vi "创建数据表.vi"(8 "error in (no error)":errorcluster) -> (0 "error out":errorcluster)   [LabVIEW 2016, in "数据查询.lvlib"]
uses:
  <vilib>/addons/database/Auxilliary.llb/DB Tools Column Info.ctl
  <vilib>/addons/database/Auxilliary.llb/DB Tools DataTypes.ctl
  <vilib>/addons/database/Connection.llb/DB Tools Open Connec (String).vi
  <userlib>/_LVST/sqlite_api/Core/Tables/SQLite_Drop Table.vi
  <userlib>/_LVST/sqlite_api/Core/Tables/SQLite_Create Table.vi
  <vilib>/addons/database/NI_Database_API.lvlib
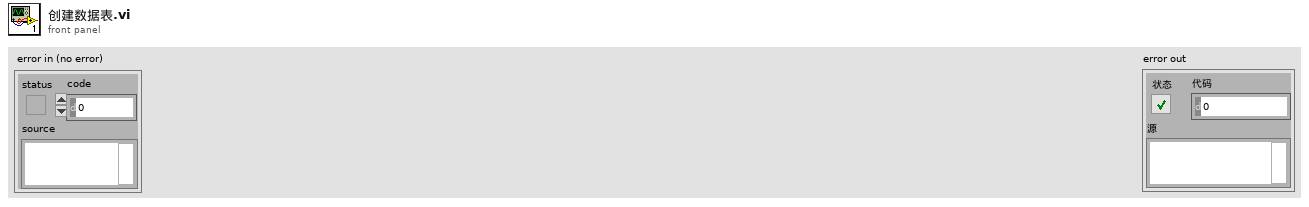
[diagram p1: front panel]
types:
  T1 = typedef "数据库类型.ctl" = enum16{"Access", "SQLite"}
  T2 = typedef "NI_Database_API.lvlib/DB Tools Column Info.ctl" = cluster{"column name":string, "data type":T3, "size":i32, "allow null?":bool}
  T3 = typedef "NI_Database_API.lvlib/DB Tools DataTypes.ctl" = enum16{"String", "Long (I32)", "Single (SGL)", "Double (DBL)", "Date/Time", "Binary"}
  T4 = typedef "NI_Database_API.lvlib/Conn ObjectReference.ctl" = refnum<k1>
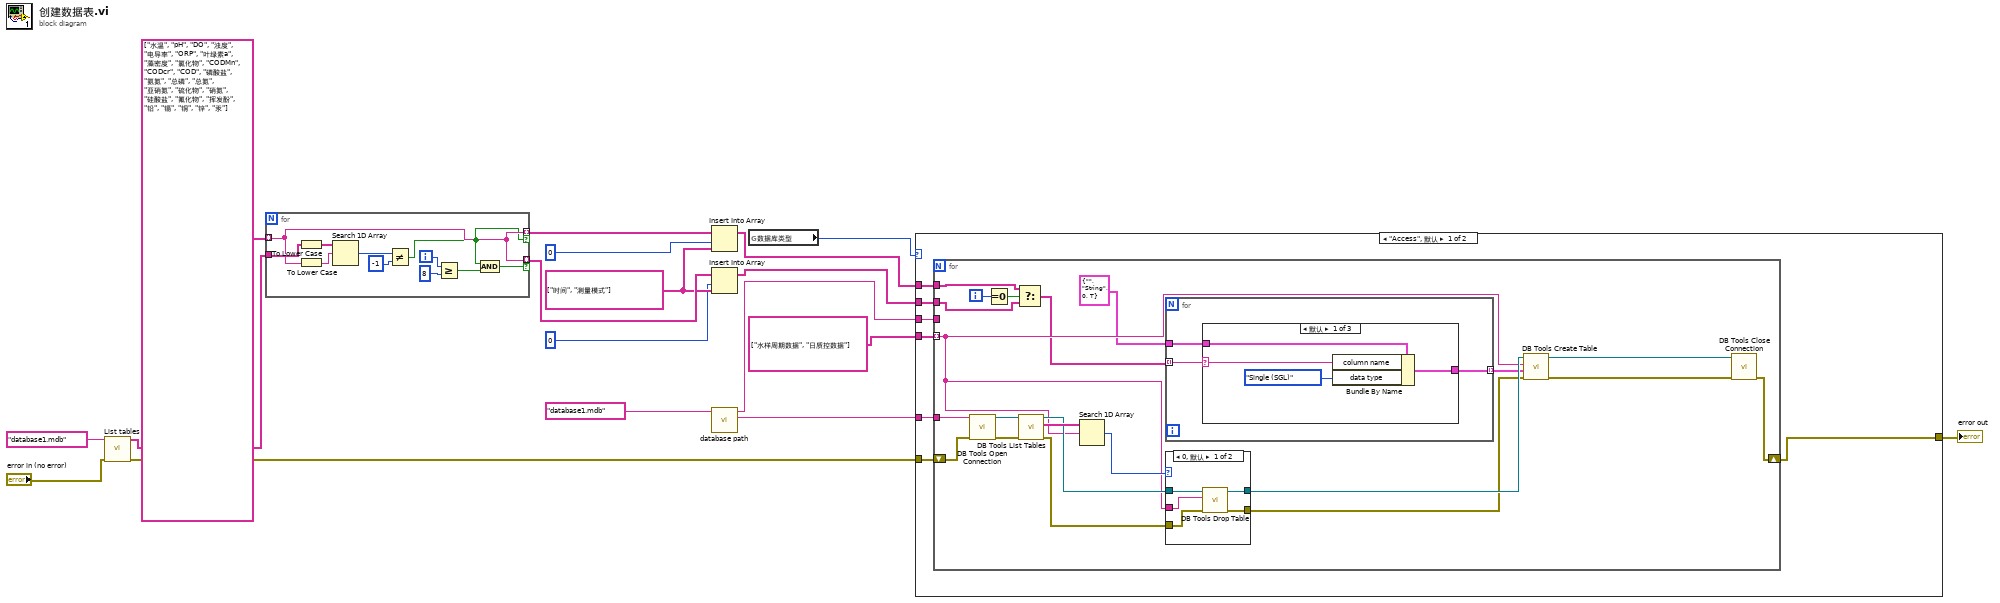
[diagram p0: block diagram]
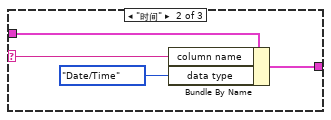
[diagram p2: hidden frame]
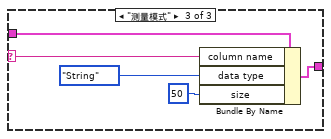
[diagram p3: hidden frame]
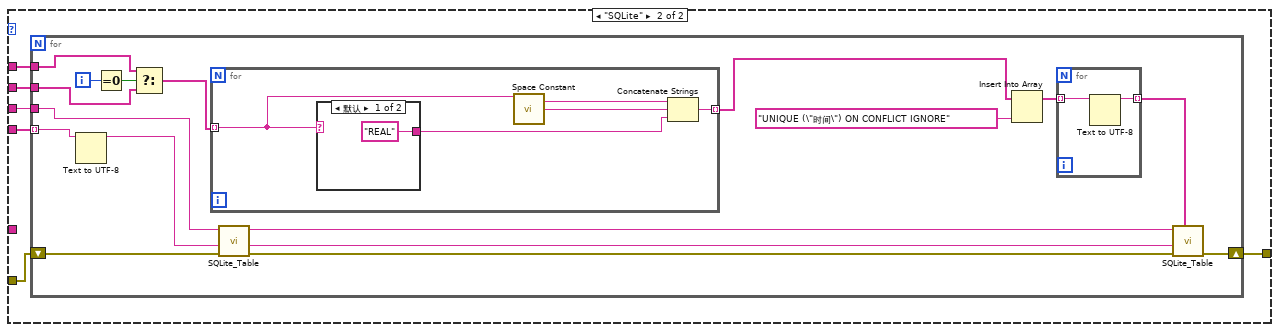
[diagram p5: hidden frame]
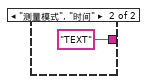
[diagram p6: hidden frame]
diagram:
  w13 = string[] ["时间", "测量模式"]
  n1 = call "List tables.vi"("error in (no error)"="error in (no error)", "database"="database1.mdb") -> ("error out"=w10:errorcluster, "tables"=w18:string[])  [unwired: 8 in]
  n2 = for {
    tunnel: string[] ["水温", "pH", "DO", "浊度", "电导率", "ORP", "叶绿素a", "藻密度", "氯化物", "CODMn", "CODcr", "COD", "磷酸盐", "氨氮", "总磷", "总氮", "亚硝氮", "硫化物", "硝氮", "硅酸盐", "氟化物", "挥发酚", "铅", "镉", "铜", "锌", "汞"] -> [w26] mode=indexing
    tunnel: w18 -> [w29]
    tunnel: [w26] -> w17 mode=indexing if=w21
    tunnel: [w26] -> w14 mode=indexing if=w22
    i -> [w25]
    n3 = To Lower Case(string=w29) -> (all lower case string=w20:string[])
    n4 = To Lower Case(string=w26) -> (all lower case string=w19:string)
    n5 = Search 1D Array(1D array=w20, element=w19) -> (index of element=w28:i32)  [unwired: 1 in]
    n6 = Not Equal?(x=w28, y=-1 ("x")) -> (x != y?=w21:bool)
    n7 = Greater Or Equal?(x=w25, y=8) -> (x >= y?=w23:bool)
    n8 = And(x=w21, y=w23) -> (x .and. y?=w22:bool)
  }
  n9 = Insert Into Array(array=w17, index=0 ("索引"), new element=w13) -> (w9:string[])
  n10 = Insert Into Array(array=w14, index=0 ("索引"), new element=w13) -> (w7:string[])
  n11 = call "database path.vi"("database"="database1.mdb") -> ("Connection information"=w2:string, "Path out"=w3:string)  [unwired: 9 in]
  n12 = global read "外部调用接口全局变量.vi" "数据库类型"() -> (w1:T1)
  n13 = case shown="\"Access\", 默认" w1 {
    tunnel: w9 -> [w36 w85]
    tunnel: w10 -> [w35 w82]
    tunnel: [w34 w83] -> w5
    tunnel: string[] ["水样周期数据", "日质控数据"] -> [w33 w86]
    tunnel: w7 -> [w32 w84]
    tunnel: w3 -> [w31 w81]
    tunnel: w2 -> [w30 _]
    frame "Access", Default {
      n14 = for {
        tunnel: w36 -> [w41]
        shift-right: [w45] -> w34
        shift-left: w35 -> [w46]
        tunnel: w33 -> [w44] mode=indexing
        tunnel: w32 -> [w40]
        tunnel: w31 -> [_]
        tunnel: w30 -> [w38]
        i -> [w43]
        n15 = call-poly <vilib>:"DB Tools Open Connection.vi"("error in (no error)"=w46, "connection information"=w38) -> ("error out"=w57:errorcluster, "connection reference"=w56:T4)  [unwired: 6 in]
        n16 = Equal To 0?(x=w43) -> (x = 0?=w42:bool)
        n17 = Select(t=w41, s=w42, f=w40) -> (s? t:f=w39:string[])
        n18 = call <vilib>:"DB Tools List Tables.vi"("error in (no error)"=w57, "connection reference"=w56) -> ("error out"=w51:errorcluster, "tables"=w55:string[], "connection reference out"=w53:T4)  [unwired: 3 in]
        n19 = Search 1D Array(1D array=w55, element=w44) -> (index of element=w54:i32)  [unwired: 1 in]
        n20 = for {
          tunnel: w39 -> [w60] mode=indexing
          tunnel: T2 {"column name"="", "data type"=enum."String", "size"=0, "allow null?"=TRUE} ("column information") -> [w59]
          tunnel: [w58] -> w47 mode=indexing
          n21 = case shown="默认" w60 {
            selector: w60 -> [w63 w67 w72]
            tunnel: w59 -> [w64 w68 w73]
            tunnel: [w62 w66 w71] -> w58
            frame Default {
              n22 = Bundle By Name(cluster=w64, "column name"=w63, "data type"=DB_Tools_DataTypes."Single (SGL)") -> (w62:T2)
            }
            frame "时间" {
              n23 = Bundle By Name(cluster=w68, "column name"=w67, "data type"=DB_Tools_DataTypes."Date/Time") -> (w66:T2)
            }
            frame "测量模式" {
              n24 = Bundle By Name(cluster=w73, "column name"=w72, "data type"=DB_Tools_DataTypes."String", "size"=50) -> (w71:T2)
            }
          }
        }
        n25 = case shown="0, 默认" w54 {
          tunnel: w53 -> [w78 w80]
          tunnel: [w77 w80] -> w52
          tunnel: w51 -> [w76 w79]
          tunnel: [w75 w79] -> w50
          tunnel: w44 -> [w74 _]
          frame 0, Default {
            n26 = call <vilib>:"DB Tools Drop Table.vi"("error in (no error)"=w76, "table"=w74, "connection reference"=w78) -> ("error out"=w75:errorcluster, "connection reference out"=w77:T4)  [unwired: 5 in]
          }
          frame -1 {
          }
        }
        n27 = call <vilib>:"DB Tools Create Table.vi"("error in (no error)"=w50, "column information"=w47, "table"=w44, "connection reference"=w52) -> ("error out"=w48:errorcluster, "connection reference out"=w49:T4)  [unwired: 4 in]
        n28 = call <vilib>:"DB Tools Close Connection.vi"("error in (no error)"=w48, "connection reference"=w49) -> ("error out"=w45:errorcluster)  [unwired: 5 in]
      }
    }
    frame "SQLite" {
      n29 = for {
        tunnel: w81 -> [w91]
        tunnel: w86 -> [w90] mode=indexing
        tunnel: w85 -> [w98]
        tunnel: w84 -> [w97]
        shift-right: [w95] -> w83
        shift-left: w82 -> [w94]
        i -> [w100]
        n30 = Text to UTF-8(11:w90) -> (3:w89:string)  [unwired: 2 in, 1 out]
        n31 = Equal To 0?(x=w100) -> (x = 0?=w99:bool)
        n32 = Select(t=w98, s=w99, f=w97) -> (s? t:f=w96:string[])
        n33 = for {
          tunnel: w96 -> [w109] mode=indexing
          tunnel: [w106] -> w92 mode=indexing
          n34 = case shown="默认" w109 {
            tunnel: ["REAL" "TEXT"] -> w107
            frame Default {
            }
            frame "测量模式", "时间" {
            }
          }
          n35 = call <vilib>:"Space Constant.vi"() -> ("String"=w108:string)
          n36 = Concatenate Strings(w109, w108, w107) -> (w106:string)
        }
        n37 = call-poly <userlib>:"SQLite_Table.vi"("DB Path"=w91, "Table Name"=w89, "error in (no error)"=w94) -> ("DB Path Out"=w103:string, "Table Name Out"=w101:string, "error out"=w102:errorcluster)  [unwired: 5 in]
        n38 = Insert Into Array(array=w92, new element="UNIQUE (\"时间\") ON CONFLICT IGNORE" ("新元素/子数组")) -> (w88:string[])  [unwired: 1 in]
        n39 = for {
          tunnel: w88 -> [w105] mode=indexing
          tunnel: [w104] -> w87 mode=indexing
          n40 = Text to UTF-8(11:w105) -> (3:w104:string)  [unwired: 2 in, 1 out]
        }
        n41 = call-poly <userlib>:"SQLite_Table.vi"("DB Path"=w103, "Table Name"=w101, "error in (no error)"=w102, "Columns"=w87) -> ("error out"=w95:errorcluster)  [unwired: 4 in, 2 out]
      }
    }
  }
  "error out" <- w5
